vi "Delete_Dots(X,Y)_Matrix-1.vi"(1 "# Frame":i32, 2 "# Dot":i32, 3 "(X,Y) IN":dbl[][](array[numeric])) -> (0 "(X,Y) OUT":dbl[][](array[numeric]))   [LabVIEW 2013]
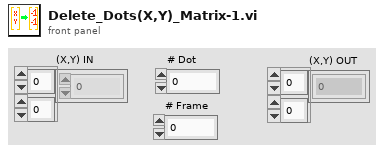
[diagram p1: front panel]
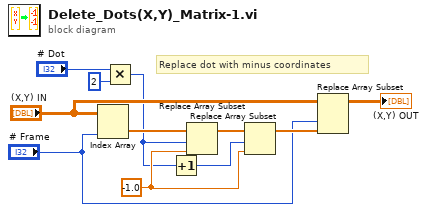
[diagram p0: block diagram]
diagram:
  w10 = -1.0 ("new element/subarray")
  # "Replace dot with minus coordinates"
  n1 = Index Array(array="(X,Y) IN", index (col)="# Frame") -> (element=w9:dbl[])  [unwired: 1 in]
  n2 = Multiply(x="# Dot", y=2) -> (x*y=w1:i32)
  n3 = Increment(x=w1) -> (x+1=w11:i32)
  n4 = Replace Array Subset(array=w9, new element=w10, index=w1) -> (w8:dbl[])
  n5 = Replace Array Subset(array=w8, new element=w10, index=w11) -> (w6:dbl[])
  n6 = Replace Array Subset(array="(X,Y) IN", new element=w6, index (col)="# Frame") -> (→"(X,Y) OUT":dbl[][])  [unwired: 1 in]
